vi "Z900_navX_SERIAL_ValidatePacketChecksum.vi"(1 "Expected Packet Length":i32, 2 "Buffer":string) -> (0 "Packet Valid":bool)   [LabVIEW 2017, in "navX Library v2.lvlib"]
uses:
  navX Library v2.lvlib
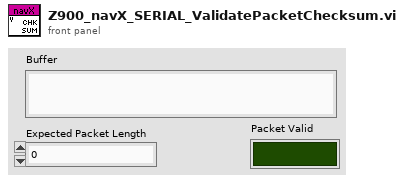
[diagram p1: front panel]
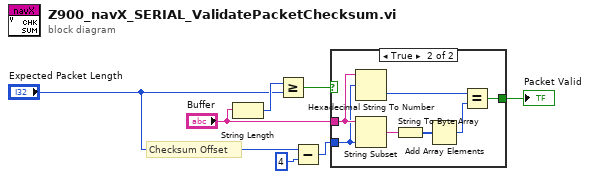
[diagram p0: block diagram]
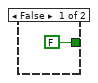
[diagram p2: hidden frame]
diagram:
  # "Checksum Offset"
  n1 = String Length(string="Buffer") -> (length=w7:i32)
  n2 = Greater Or Equal?(x=w7, y="Expected Packet Length") -> (x >= y?=w4:bool)
  n3 = Subtract(x="Expected Packet Length", y=4) -> (x-y=w3:i32)
  n4 = case shown="True" w4 {
    tunnel: w3 -> [_ w12]
    tunnel: [FALSE w9] -> w2
    tunnel: "Buffer" -> [_ w13]
    frame False {
    }
    frame True {
      n5 = Hexadecimal String To Number(string=w13, offset=w12) -> (number=w10:u32)  [unwired: 1 in, 1 out]
      n6 = String Subset(string=w13, length (rest)=w12) -> (substring=w15:string)  [unwired: 1 in]
      n7 = String To Byte Array(string=w15) -> (unsigned byte array=w14:u8[])
      n8 = Add Array Elements(numeric array=w14) -> (sum=w11:u8)
      n9 = Equal?(x=w10, y=w11) -> (x = y?=w9:bool)
    }
  }
  "Packet Valid" <- w2
